vi "Set.vi"(8 "error in (no error)":errorcluster, 10 "Numeric":dbl, 11 "Instrument in":refnum<class "Instrument.lvclass">) -> (0 "error out":errorcluster, 3 "Instrument out":refnum<class "Instrument.lvclass">)   [LabVIEW 2014, in "Instrument.lvclass"]
uses:
  Instrument.lvclass
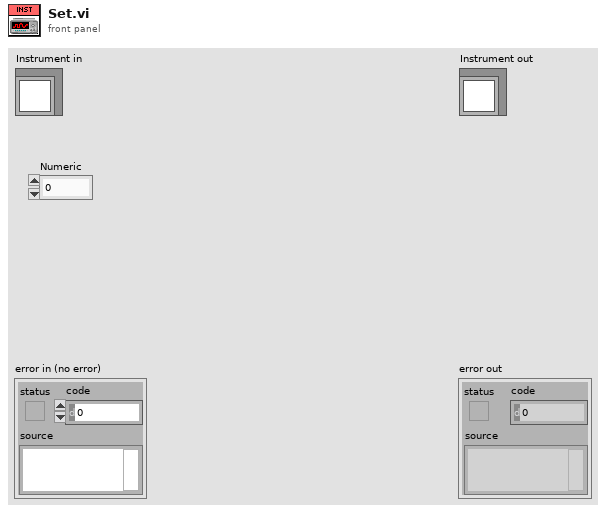
[diagram p1: front panel]
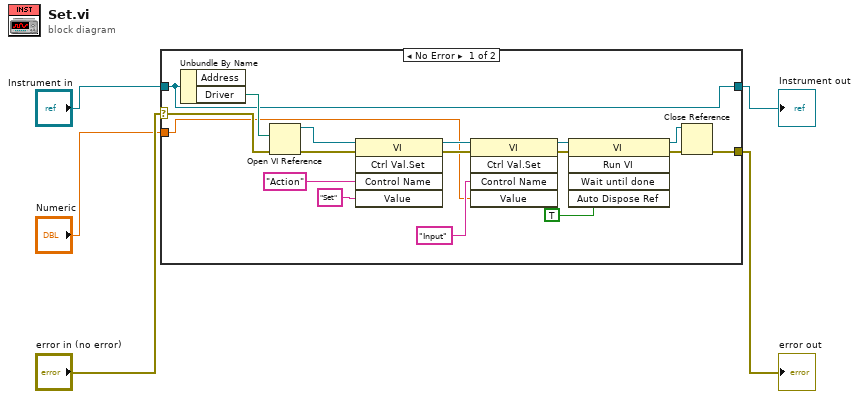
[diagram p0: block diagram]
diagram:
  n1 = case shown="No Error" "error in (no error)" {
    selector: "error in (no error)" -> [w19 w24]
    tunnel: [w7 w24] -> w4
    tunnel: [w18 w23] -> w2
    tunnel: "Instrument in" -> [w18 w23]
    tunnel: "Numeric" -> [w12 _]
    frame No Error {
      n2 = Unbundle By Name(w18) -> ("Driver"=w22:path)  [unwired: 1 out]
      n3 = Open VI Reference(vi path=w22, error in (no error)=w19) -> (vi reference=w14:refnum<vi>, error out=w16:errorcluster)  [unwired: 4 in]
      n4 = invoke class="VI" method="Ctrl Val.Set"(reference=w14, error in=w16, "Control Name"="Action", "Value"="Set" ("Control Name")) -> (reference out=w17:refnum<vi>, error out=w15:errorcluster)  [unwired: 1 in, 3 out]
      n5 = invoke class="VI" method="Ctrl Val.Set"(reference=w17, error in=w15, "Control Name"="Input", "Value"=w12) -> (reference out=w11:refnum<vi>, error out=w9:errorcluster)  [unwired: 1 in, 3 out]
      n6 = invoke class="VI" method="Run VI"(reference=w11, error in=w9, "Wait until done"=TRUE ("Wait Until Done")) -> (reference out=w10:refnum<vi>, error out=w8:errorcluster)  [unwired: 2 in, 3 out]
      n7 = Close Reference(reference=w10, error in (no error)=w8) -> (error out=w7:errorcluster)
    }
    frame Error {
    }
  }
  "error out" <- w4
  "Instrument out" <- w2
